vi "dfd_Super Narrowband Filter Design Specification Conversion.vi"(6 "fs [Hz]":dbl=1.0 format="%.2f", 7 "filter type":T2(ring), 8 "error in (no error)":errorcluster, 11 "freq specs [Hz]":T1) -> (0 "error out":errorcluster, 1 "fc":dbl, 2 "fstop":dbl, 3 "fpass":dbl)   [LabVIEW 2017, in "NI_DigFilter_Process.lvlib"]
doc: "Converts the classical filter design specification to super narrowband filter design specification."
uses:
  <vilib>/addons/Digital Filter Design/NI_DigFilter_Process.lvlib
  <vilib>/addons/Digital Filter Design/_Objects.llb/DFD Filter Frequence Specification (Design).ctl
  <vilib>/addons/Digital Filter Design/NI_DigFilterLicensed.lvlib
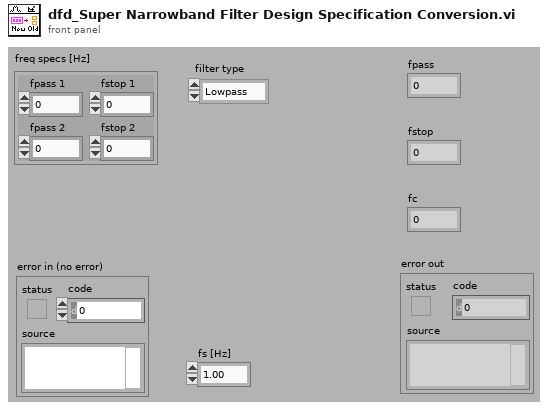
[diagram p1: front panel]
types:
  T1 = typedef "NI_DigFilterLicensed.lvlib/DFD Filter Frequence Specification (Design).ctl" = cluster{"fpass 1":dbl, "fstop 1":dbl, "fpass 2 ":dbl, "fstop 2":dbl}
  T2 = enum16{"Lowpass", "Highpass", "Bandpass", "Bandstop"}
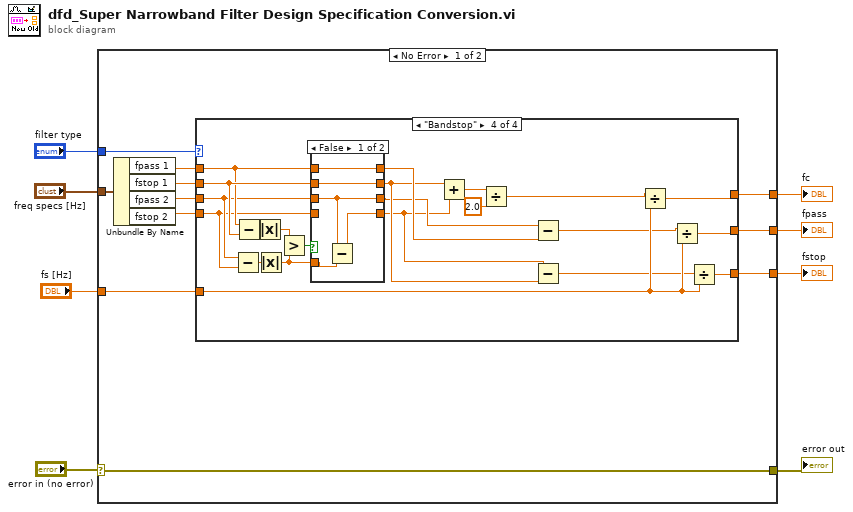
[diagram p0: block diagram]
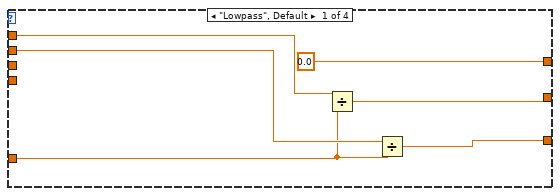
[diagram p2: hidden frame]
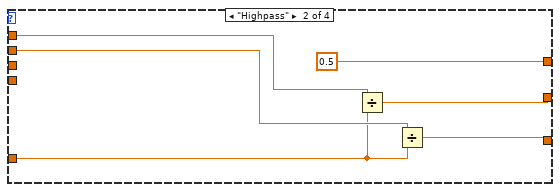
[diagram p3: hidden frame]
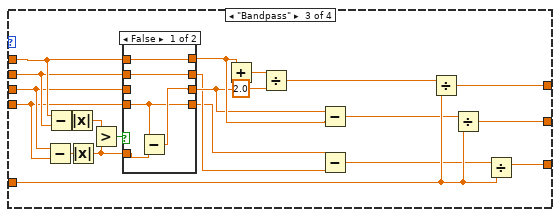
[diagram p4: hidden frame]
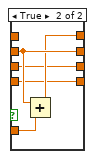
[diagram p5: hidden frame]
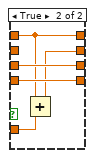
[diagram p6: hidden frame]
diagram:
  n1 = case shown="No Error" "error in (no error)" {
    selector: "error in (no error)" -> [w9 w96]
    tunnel: "filter type" -> [w19 _]
    tunnel: "freq specs [Hz]" -> [w18 _]
    tunnel: [w17 _] -> w6
    tunnel: [w16 _] -> w5
    tunnel: [w15 _] -> w4
    tunnel: "fs [Hz]" -> [w10 _]
    tunnel: [w9 w96] -> w1
    frame No Error {
      n2 = Unbundle By Name(w18) -> ("fpass 1"=w14:dbl, "fstop 1"=w13:dbl, "fpass 2"=w12:dbl, "fstop 2"=w11:dbl)
      n3 = case shown="\"Bandstop\"" w19 {
        tunnel: w14 -> [w23 w29 w45 w78]
        tunnel: w13 -> [w21 w27 w44 w79]
        tunnel: w12 -> [_ _ w43 w77]
        tunnel: w11 -> [_ _ w42 w76]
        tunnel: [0.0 0.5 w37 w69] -> w17
        tunnel: [w24 w30 w36 w66] -> w16
        tunnel: [w22 w28 w34 w67] -> w15
        tunnel: w10 -> [w20 w26 w35 w68]
        frame "Lowpass", Default {
          n4 = Divide(x=w23, y=w20) -> (x/y=w24:dbl)
          n5 = Divide(x=w21, y=w20) -> (x/y=w22:dbl)
        }
        frame "Highpass" {
          n6 = Divide(x=w29, y=w26) -> (x/y=w30:dbl)
          n7 = Divide(x=w27, y=w26) -> (x/y=w28:dbl)
        }
        frame "Bandpass" {
          n8 = Subtract(x=w43, y=w42) -> (x-y=w47:dbl)
          n9 = Subtract(x=w45, y=w44) -> (x-y=w46:dbl)
          n10 = Absolute Value(x=w46) -> (abs(x)=w48:dbl)
          n11 = Absolute Value(x=w47) -> (abs(x)=w50:dbl)
          n12 = Greater?(x=w48, y=w50) -> (0:w49:bool)
          n13 = case shown="False" w49 {
            tunnel: w44 -> [w57 w63]
            tunnel: w45 -> [w58 _]
            tunnel: w43 -> [_ w60]
            tunnel: w42 -> [w54 w59]
            tunnel: [w57 w63] -> w39
            tunnel: w50 -> [w56 w62]
            tunnel: [w58 w61] -> w41
            tunnel: [w55 w60] -> w40
            tunnel: [w54 w59] -> w38
            frame False {
              n14 = Subtract(x=w54, y=w56) -> (x-y=w55:dbl)
            }
            frame True {
              n15 = Add(x=w63, y=w62) -> (x+y=w61:dbl)
            }
          }
          n16 = Add(x=w41, y=w40) -> (x+y=w53:dbl)
          n17 = Divide(x=w53, y=2.0) -> (x/y=w51:dbl)
          n18 = Subtract(x=w40, y=w41) -> (x-y=w33:dbl)
          n19 = Subtract(x=w38, y=w39) -> (x-y=w32:dbl)
          n20 = Divide(x=w51, y=w35) -> (x/y=w37:dbl)
          n21 = Divide(x=w33, y=w35) -> (x/y=w36:dbl)
          n22 = Divide(x=w32, y=w35) -> (x/y=w34:dbl)
        }
        frame "Bandstop" {
          n23 = Subtract(x=w77, y=w76) -> (x-y=w82:dbl)
          n24 = Subtract(x=w78, y=w79) -> (x-y=w83:dbl)
          n25 = Absolute Value(x=w83) -> (abs(x)=w81:dbl)
          n26 = Absolute Value(x=w82) -> (abs(x)=w75:dbl)
          n27 = Greater?(x=w81, y=w75) -> (0:w80:bool)
          n28 = case shown="False" w80 {
            tunnel: w79 -> [w89 _]
            tunnel: w78 -> [w90 w91]
            tunnel: w77 -> [w87 w94]
            tunnel: w76 -> [_ w93]
            tunnel: [w89 w92] -> w73
            tunnel: w75 -> [w88 w95]
            tunnel: [w90 w91] -> w74
            tunnel: [w87 w94] -> w72
            tunnel: [w86 w93] -> w71
            frame False {
              n29 = Subtract(x=w87, y=w88) -> (x-y=w86:dbl)
            }
            frame True {
              n30 = Add(x=w91, y=w95) -> (x+y=w92:dbl)
            }
          }
          n31 = Add(x=w73, y=w71) -> (x+y=w84:dbl)
          n32 = Divide(x=w84, y=2.0) -> (x/y=w70:dbl)
          n33 = Subtract(x=w72, y=w74) -> (x-y=w65:dbl)
          n34 = Subtract(x=w71, y=w73) -> (x-y=w64:dbl)
          n35 = Divide(x=w70, y=w68) -> (x/y=w69:dbl)
          n36 = Divide(x=w65, y=w68) -> (x/y=w66:dbl)
          n37 = Divide(x=w64, y=w68) -> (x/y=w67:dbl)
        }
      }
    }
    frame Error {
    }
  }
  "fc" <- w6
  "fpass" <- w5
  "fstop" <- w4
  "error out" <- w1
